vi "svfa_Average Array (real) No State_spectrum state.vi"(6 "previous avg real spectrum":cluster{"f0":dbl, "df":dbl, "real FFT":dbl[]} {"real FFT" format="%.2f"; "df" format="%.2f"; "f0" format="%.2f"}, 7 "processing control":T1(ring), 8 "averages completed":dbl format="%.2f", 9 "averaging parameters":T2={"averaging mode"=enum."No averaging", "weighting mode"=enum."Linear", "number of averages"=10, "linear mode"=enum."Auto restart"}, 11 "array":dbl[](array[numeric]) format="%.2f") -> (0 "averages completed":dbl, 1 "averaging done":bool, 4 "new avg real spectrum":cluster{"f0":dbl, "df":dbl, "real FFT":dbl[]} {"real FFT" format="%.2f"; "df" format="%.2f"; "f0" format="%.2f"})   [LabVIEW 2017]
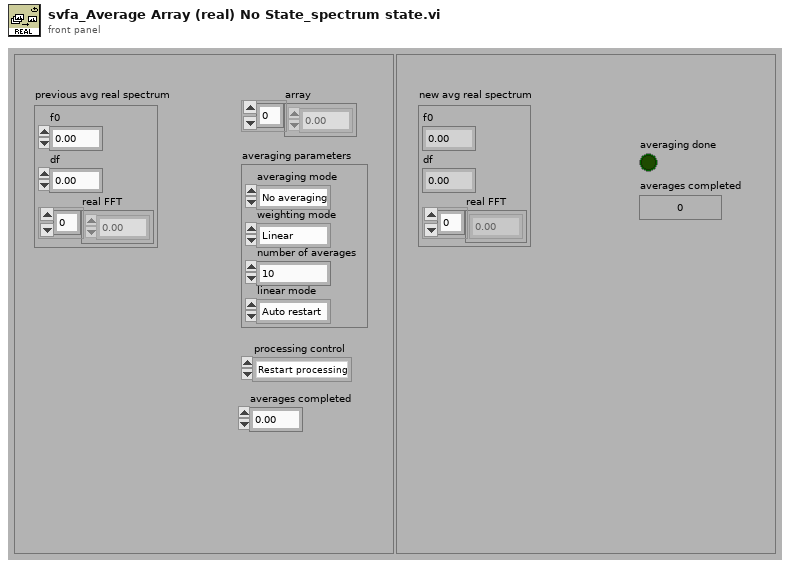
[diagram p1: front panel]
types:
  T1 = enum16{"Restart processing", "Continue processing", "Skip processing"}
  T2 = cluster{"averaging mode":enum16{"No averaging", "Vector averaging", "RMS averaging", "Peak hold"}, "weighting mode":enum16{"Linear", "Exponential"}, "number of averages":u32, "linear mode":enum16{"One shot", "Auto restart"}}
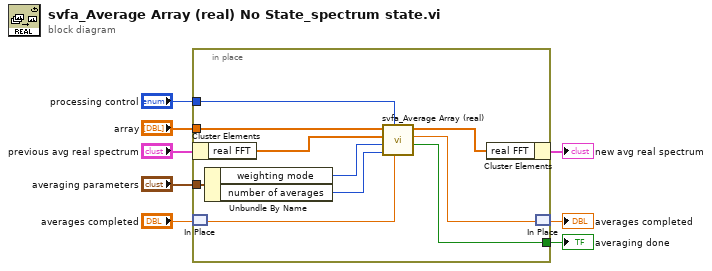
[diagram p0: block diagram]
diagram:
  n1 = in-place {
    in-place-border: "array" -> [w18]
    in-place-border: [w17] -> w7
    in-place-border: "processing control" -> [w14]
    in-place-border: "averaging parameters" -> [w13]
    n2 = in-place-cluster #1("previous avg real spectrum") -> ("real FFT"=w12:dbl[])
    n3 = in-place-match #2("averages completed") -> (w10:dbl)
    n4 = Unbundle By Name(w13) -> ("weighting mode"=w16:enum16{"Linear", "Exponential"}, "number of averages"=w15:u32)
    n5 = call <vilib>:"svfa_Average Array (real).vi"("averages completed in"=w10, "processing control"=w14, "number of averages"=w15, "weighting mode"=w16, "previous average array"=w12, "array"=w18) -> ("averaging done"=w17:bool, "averages completed out"=w9:dbl, "average array"=w11:dbl[])  [unwired: 3 in]
    n6 = in-place-cluster #1("real FFT"=w11) -> (→"new avg real spectrum":cluster{"f0":dbl, "df":dbl, "real FFT":dbl[]})
    n7 = in-place-match #2(w9) -> (→"averages completed":dbl)
  }
  "averaging done" <- w7
